vi "Wait for Data.vi"(8 "error in (no error)":errorcluster, 11 "Pulse Recorder in":refnum<class "Pulse Recorder.lvclass">) -> (0 "error out":errorcluster, 3 "Pulse Recorder out":refnum<class "Pulse Recorder.lvclass">)   [LabVIEW 2015, in "Pulse Recorder.lvclass"]
uses:
  Pulse Recorder.lvclass
  Pulse Recorder.lvclass/Pulse Recorder.ctl
  Measure Object/Measure Object.lvclass/Measure Object.ctl
  Measure Object Messages/Self-Addressed Msg/Self-addressed Msg.lvclass/Self-addressed Msg.ctl
  Pulse Controller Messages/Armed Response Msg/Armed Response Msg.lvclass/Armed Response Msg.ctl
  <vilib>/ActorFramework/Message Enqueuer/Message Enqueuer.lvclass/Message Enqueuer.ctl
  Results/Acquired Result/Acquired Result.lvclass/Acquired Result.ctl
  <vilib>/ActorFramework/Actor/Actor.lvclass/Actor.ctl
  Measure Object/Read Name.vi
  Measure Object/Read Reply to.vi
  Measure Object Messages/Self-Addressed Msg/Read Return Enqueuer.vi
  Results/Acquired Result/Read Finished.vi
  Results/Acquired Result/Write Sender.vi
  <vilib>/ActorFramework/Message Enqueuer/Enqueue.vi
  <vilib>/ActorFramework/Message Enqueuer/Init from Existing Queue.vi
  <vilib>/ActorFramework/Message Priority Queue/Priority Enqueue.vi
  <vilib>/ActorFramework/Time-Delayed Send Message/Time-Delayed Send Message.vi
  Measure Object Messages/Result Reply Msg/Result Reply Msg.lvclass
  <vilib>/ActorFramework/Message Enqueuer/Message Enqueuer.lvclass
  Pulse Controller Messages/Armed Response Msg/Armed Response Msg.lvclass
  Pulse Recorder Messages/Wait for Data Msg/Wait for Data Msg.lvclass
  <vilib>/ActorFramework/Actor/Actor.lvclass
  Results/Acquired Result/Acquired Result.lvclass
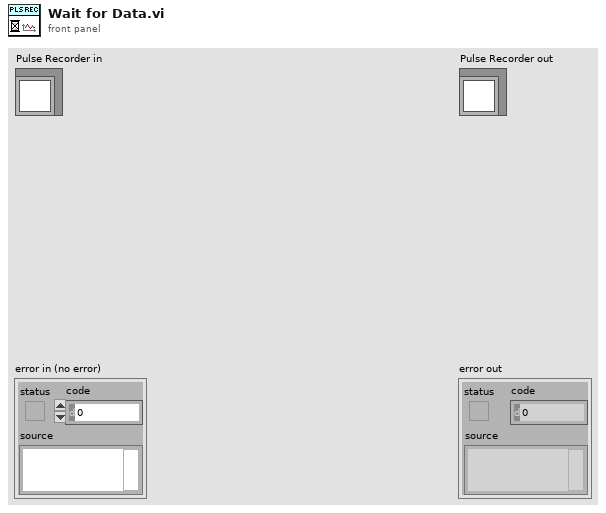
[diagram p1: front panel]
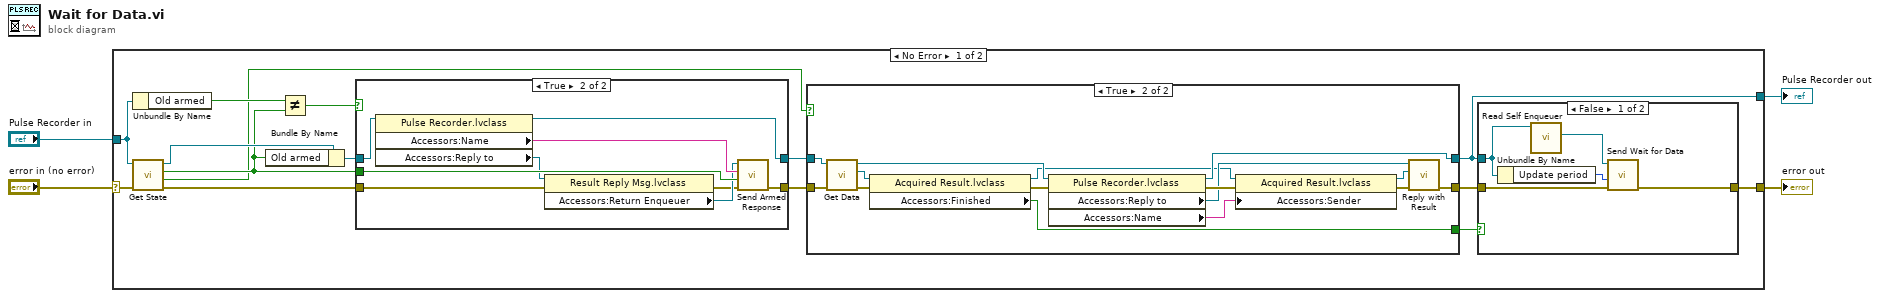
[diagram p0: block diagram]
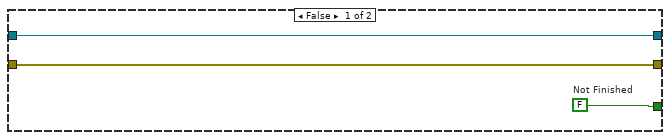
[diagram p4: hidden frame]
diagram:
  n1 = case shown="No Error" "error in (no error)" {
    selector: "error in (no error)" -> [w19 w56]
    tunnel: [w5 w56] -> w3
    tunnel: [w7 w55] -> w1
    tunnel: "Pulse Recorder in" -> [w13 w55]
    frame No Error {
      n2 = Unbundle By Name(w13) -> ("Old armed"=w18:bool)
      n3 = call-dynamic "Get State.vi"("error in (no error)"=w19, "Pulse Controller in"=w13) -> ("error out"=w16:errorcluster, "Data ready"=w9:bool, "Armed"=w10:bool, "Pulse Controller out"=w12:refnum<class "Pulse Recorder.lvclass">)  [unwired: 6 in]
      n4 = Bundle By Name(cluster=w12, "Old armed"=w10) -> (w11:refnum<class "Pulse Recorder.lvclass">)
      n5 = Not Equal?(x=w18, y=w10) -> (x != y?=w17:bool)
      n6 = case shown="True" w17 {
        tunnel: w11 -> [w26 w36]
        tunnel: w16 -> [w27 w29]
        tunnel: [w27 w34] -> w15
        tunnel: w10 -> [_ w33]
        tunnel: [w26 w32] -> w14
        frame False {
        }
        frame True {
          n7 = property class="Pulse Recorder.lvclass"(reference=w36) -> (reference out=w32:refnum<class "Pulse Recorder.lvclass">, "Accessors:Name"=w35:string, "Accessors:Reply to"=w31:refnum<class "Result Reply Msg.lvclass">)  [unwired: 1 in, 1 out]
          n8 = property class="Result Reply Msg.lvclass"(reference=w31, error in=w29) -> (error out=w28:errorcluster, "Accessors:Return Enqueuer"=w30:refnum<class "Message Enqueuer.lvclass">)  [unwired: 1 out]
          n9 = call "Send Armed Response.vi"("error in (no error)"=w28, "Armed"=w33, "Sender"=w35, "Message Enqueuer"=w30) -> ("error out"=w34:errorcluster)  [unwired: 6 in, 1 out]
        }
      }
      n10 = case shown="True" w9 {
        tunnel: w14 -> [w39 w54]
        tunnel: w15 -> [w38 w52]
        tunnel: [w38 w44] -> w6
        tunnel: [w39 w51] -> w7
        tunnel: [w37 w40] -> w8
        frame False {
          w37 = FALSE  # Not Finished
        }
        frame True {
          n11 = call-dynamic "Get Data.vi"("error in (no error)"=w52, "Pulse Recorder in"=w54) -> ("error out"=w42:errorcluster, "Data Result"=w50:refnum<class "Acquired Result.lvclass">, "Pulse Recorder out"=w53:refnum<class "Pulse Recorder.lvclass">)  [unwired: 7 in]
          n12 = property class="Acquired Result.lvclass"(reference=w50, error in=w42) -> (reference out=w43:refnum<class "Acquired Result.lvclass">, error out=w41:errorcluster, "Accessors:Finished"=w40:bool)
          n13 = property class="Pulse Recorder.lvclass"(reference=w53, error in=w41) -> (reference out=w51:refnum<class "Pulse Recorder.lvclass">, error out=w49:errorcluster, "Accessors:Reply to"=w47:refnum<class "Result Reply Msg.lvclass">, "Accessors:Name"=w48:string)
          n14 = property class="Acquired Result.lvclass"(reference=w43, error in=w49, "Accessors:Sender"=w48) -> (reference out=w46:refnum<class "Acquired Result.lvclass">, error out=w45:errorcluster)
          n15 = call-dynamic "Reply with Result.vi"("error in (no error)"=w45, "Result"=w46, "Result Reply Msg in"=w47) -> ("error out"=w44:errorcluster)  [unwired: 7 in, 1 out]
        }
      }
      n16 = case shown="False" w8 {
        tunnel: w7 -> [w20 _]
        tunnel: w6 -> [w22 w25]
        tunnel: [w21 w25] -> w5
        frame False {
          n17 = Unbundle By Name(w20) -> ("Update period"=w23:i32)
          n18 = call <vilib>:"Read Self Enqueuer.vi"("Actor"=w20) -> ("Self Enqueuer"=w24:refnum<class "Message Enqueuer.lvclass">)  [unwired: 10 in]
          n19 = call "Send Wait for Data.vi"("error in (no error)"=w22, "Milliseconds To Wait"=w23, "Message Enqueuer"=w24) -> ("error out"=w21:errorcluster)  [unwired: 6 in, 2 out]
        }
        frame True {
        }
      }
    }
    frame Error {
    }
  }
  "error out" <- w3
  "Pulse Recorder out" <- w1
